vi "Helper - NoSailZone to Log String.vi"(9 "Global No Sail Circles":T1[](array[typedef]), 10 "Selector":string, 11 "PrevString":string) -> (3 "Output":string)   [LabVIEW 2011]
doc: "Part of Helper - Data to String.vi. Look there for more details."
uses:
  2 Typedefs/UTM Circle.ctl
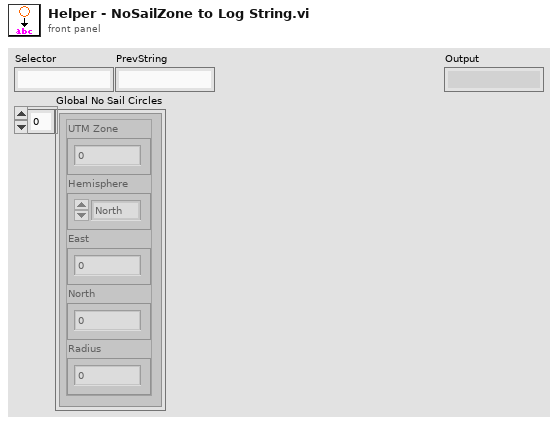
[diagram p1: front panel]
types:
  T1 = typedef "UTM Circle.ctl" = cluster{"UTM Zone":dbl, "Hemisphere":enum16{"North", "South"}, "East":dbl, "North":dbl, "Radius":dbl}
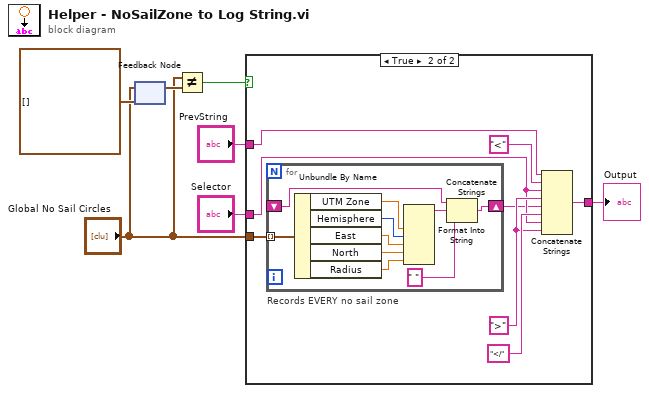
[diagram p0: block diagram]
diagram:
  n1 = feedback #1(T1[] [] ("Global No Sail Circles")) -> (w5:T1[])
  n2 = feedback-in #1("Global No Sail Circles") -> ()
  n3 = Not Equal?(x="Global No Sail Circles", y=w5) -> (x != y?=w1:bool)
  n4 = case shown="True" w1 {
    tunnel: [w8 w16] -> w6
    tunnel: "Selector" -> [_ w11]
    tunnel: "Global No Sail Circles" -> [_ w9]
    tunnel: "PrevString" -> [w8 w12]
    frame False {
    }
    frame True {
      w13 = ">" ("string")
      n5 = for "Records EVERY no sail zone" {
        tunnel: w9 -> [w26] mode=indexing
        shift-right: [w19] -> w10
        shift-left: _ -> [w18]
        n6 = Unbundle By Name(w26) -> ("UTM Zone"=w25:dbl, "Hemisphere"=w24:enum16{"North", "South"}, "East"=w23:dbl, "North"=w22:dbl, "Radius"=w21:dbl)
        n7 = Format Into String(w25, w24, w23, w22, w21) -> (resulting string=w20:string)  [unwired: 3 in, 1 out]
        n8 = Concatenate Strings(w18, w20, " " ("string")) -> (w19:string)
      }
      n9 = Concatenate Strings(w12, "<" ("string"), w11, w13, w10, "</" ("string"), w11, w13) -> (w16:string)
    }
  }
  "Output" <- w6
